vi "thscan_comparator_pix25.vi"() -> ()   [LabVIEW 2022 SP3]
panel:
  in  "Tab Control":enum32{"Single", "ROI"}(tab)
  out "Th Scan":u32[][](graph)=[[1, 1, 1, 1, 1, 1, 1, 1, 2, 71, 15005, 878042, 479272, 831838, 354879, 167379, 90908, 5540, 1668, 1480, 1359, 1170, 1144, 1050, 939, 886, 809, 720, 677, 630, 576, 523, 519, 483, 437, 402, 356, 337, 307, 320, 264, 275, 227, 222, 203, 176, 182, 179, 159, 135, 121, 110, 95, 105, 99, 71, 94, 91, 67, 61, 58, 55, 48, 31, 24, 26, 23, 15, 23, 17, 9, 11, 7, 5, 5, 4, 3, 3, 3, 1, 2, 2, 0, 1, 0, 0, 1, 0, 0, 1, 1, 0, 1, 1, 0, 0, 0, 0, 0, 0, 0], [1, 1, 1, 1, 1, 1, 1, 1, 2, 113, 14536, 860293, 575187, 892530, 326807, 156931, 85898, 3891, 481, 322, 328, 309, 273, 253, 234, 196, 206, 205, 157, 166, 143, 168, 135, 110, 116, 106, 90, 92, 74, 96, 70, 63, 73, 60, 55, 53, 50, 39, 38, 43, 33, 32, 28, 28, 21, 27, 19, 19, 15, 9, 10, 10, 10, 8, 8, 7, 5, 5, 10, 8, 6, 3, 2, 2, 0, 1, 1, 1, 0, 0, 0, 1, 1, 1, 0, 0, 0, 0, 0, 1, 0, 0, 0, 0, 0, 0, 0, 0, 0, 0, 0]]
  out "ThScans_Family":u32[][](graph)
  in  "Current File":u16(ring) items=["RED", "BLUE"]
  in  "file blue":path=path "C:/Users/User/OneDrive/measurements/pix25/PIX25/17_04_2023/M1/1_CountRate_gate_1s_iKRUM_14_setting_1/TS_step_10/itube_020_0417_101556"
  in  "file red":path=path "C:/Users/User/OneDrive/measurements/pix25/PIX25/17_04_2023/M1/1_CountRate_gate_1s_iKRUM_14_setting_1/TS_step_10/itube_080_0417_100615"
  out "MainImg":u32[][](graph)
  in  "ThScan_Load":bool
  in  "Exit":bool
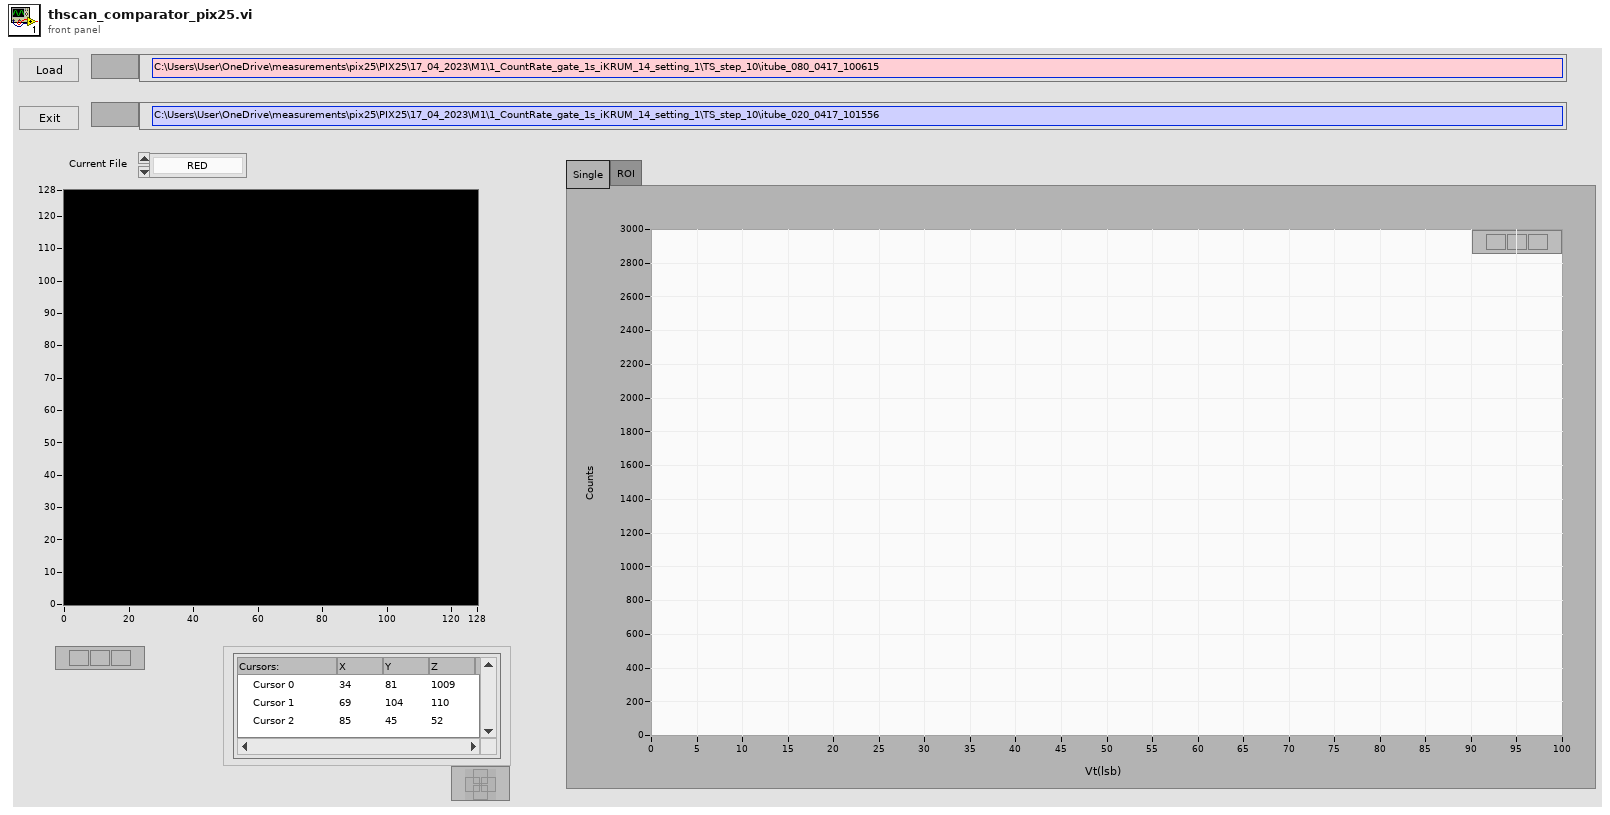
[diagram p1: front panel]
types:
  T1 = typedef "LVPointDoubleTypeDef.ctl" = cluster{"Cursor X":dbl, "Cursor Y":dbl}
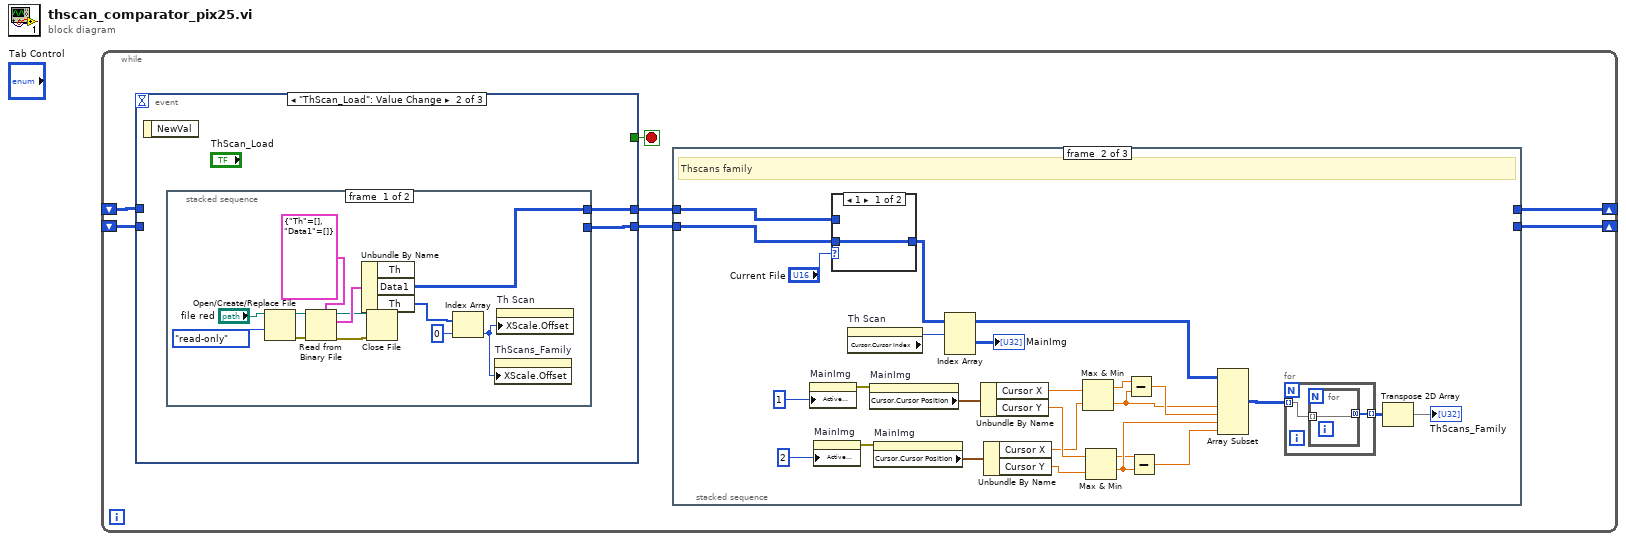
[diagram p0: block diagram]
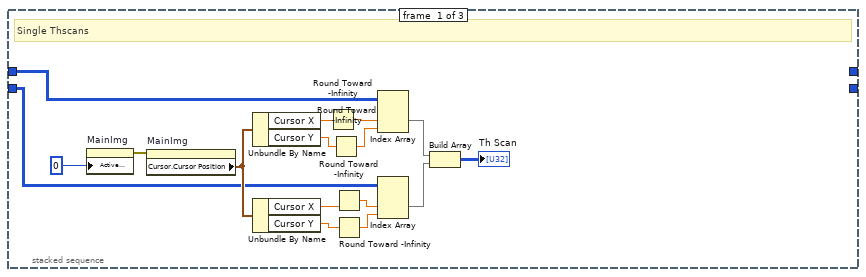
[diagram p2: hidden frame]
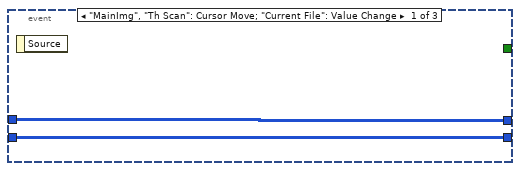
[diagram p5: hidden frame]
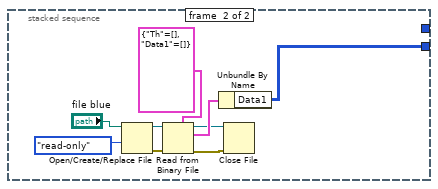
[diagram p6: hidden frame]
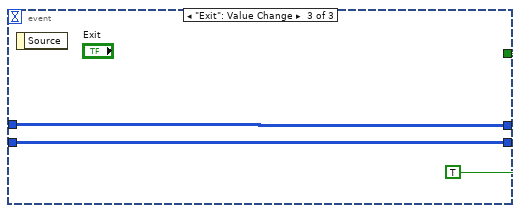
[diagram p7: hidden frame]
diagram:
  n1 = while {
    shift-right: [w1] -> _
    shift-left: _ -> [w6]
    shift-right: [w2] -> _
    shift-left: _ -> [w5]
    stop <- w7 stop-if-true
    n2 = event shown="[1] \"ThScan_Load\": Value Change" {
      selector: _ -> [_ _ _]
      dyn-events: _ -> [_ _ _]
      timeout: _ -> [_ _ _]
      tunnel: [_ _ TRUE] -> w7
      tunnel: w6 -> [w57 _ w82]
      tunnel: [w57 w59 w82] -> w4
      tunnel: [w56 w58 w81] -> w3
      tunnel: w5 -> [w56 _ w81]
      event "MainImg", "Th Scan": Cursor Move; "Current File": Value Change {
        n3 = event-data() -> ()  [unwired: 1 in, 1 out]
      }
      event "ThScan_Load": Value Change {
        n4 = event-data() -> ()  [unwired: 1 in, 1 out]
        n5 = stacked-sequence {
          tunnel: [_ w72] -> w59
          tunnel: [w60 _] -> w58
          frame #0 {
            n6 = Open/Create/Replace File(file path (use dialog)="file red", access (0:read/write)=enum16{"read/write", "read-only", "write-only"}."read-only") -> (refnum out=w68:refnum<file>, error out=w67:errorcluster)  [unwired: 4 in, 1 out]
            n7 = Read from Binary File(5:cluster{"Th":u16[], "Data1":u32[][][]} {"Th"=[], "Data1"=[]} ("TH Gate Scan"), 8:w67, 11:w68) -> (0:w70:errorcluster, 2:w71:cluster{"Th":u16[], "Data1":u32[][][]}, 3:w69:refnum<file>)  [unwired: 3 in, 1 out]
            n8 = Unbundle By Name(w71) -> ("Data1"=w60:u32[][][], "Th"=w61:u16[])  [unwired: 1 out]
            n9 = Close File(refnum=w69, error in=w70) -> ()  [unwired: 2 out]
            n10 = Index Array(array=w61, index=0) -> (element=w62:u16)
            n11 = property on="ThScans_Family" class="WFGraph (strict)"("XScale.Offset"=w62) -> ()  [unwired: 2 in, 2 out]
            n12 = property on="Th Scan" class="WFGraph (strict)"("XScale.Offset"=w62) -> ()  [unwired: 2 in, 2 out]
          }
          frame #1 {
            n13 = Open/Create/Replace File(file path (use dialog)="file blue", access (0:read/write)=enum16{"read/write", "read-only", "write-only"}."read-only") -> (refnum out=w77:refnum<file>, error out=w76:errorcluster)  [unwired: 4 in, 1 out]
            n14 = Read from Binary File(5:cluster{"Th":u16[], "Data1":u32[][][]} {"Th"=[], "Data1"=[]} ("TH Gate Scan"), 8:w76, 11:w77) -> (0:w79:errorcluster, 2:w80:cluster{"Th":u16[], "Data1":u32[][][]}, 3:w78:refnum<file>)  [unwired: 3 in, 1 out]
            n15 = Unbundle By Name(w80) -> ("Data1"=w72:u32[][][])
            n16 = Close File(refnum=w78, error in=w79) -> ()  [unwired: 2 out]
          }
        }
      }
      event "Exit": Value Change {
        n17 = event-data() -> ()  [unwired: 1 in, 1 out]
      }
    }
    n18 = stacked-sequence {
      tunnel: w4 -> [w8 w24 w54]
      tunnel: w3 -> [w9 w25 w55]
      tunnel: [_ _ w55] -> w2
      tunnel: [_ _ w54] -> w1
      frame #0 {
        # "Single Thscans"
        n19 = property on="MainImg" class="IntGraph (strict)"("Active Cursor"=u32 0) -> (error out=w11:errorcluster)  [unwired: 2 in, 1 out]
        n20 = property on="MainImg" class="IntGraph (strict)"(error in=w11) -> ("Cursor.Cursor Position"=w12:T1)  [unwired: 1 in, 2 out]
        n21 = Unbundle By Name(w12) -> ("Cursor X"=w21:dbl, "Cursor Y"=w22:dbl)
        n22 = Unbundle By Name(w12) -> ("Cursor X"=w17:dbl, "Cursor Y"=w18:dbl)
        n23 = Round Toward -Infinity(1:w21) -> (0:w20:dbl)
        n24 = Round Toward -Infinity(1:w22) -> (0:w23:dbl)
        n25 = Round Toward -Infinity(1:w17) -> (0:w16:dbl)
        n26 = Round Toward -Infinity(1:w18) -> (0:w19:dbl)
        n27 = Index Array(array=w9, index (dim 1)=w20, index (dim 2)=w23) -> (element=w15:u32[])  [unwired: 1 in]
        n28 = Index Array(array=w8, index (dim 1)=w16, index (dim 2)=w19) -> (element=w14:u32[])  [unwired: 1 in]
        n29 = Build Array(w15, w14) -> (→"Th Scan":u32[][])
      }
      frame #1 {
        # "Thscans family"
        n30 = property on="MainImg" class="IntGraph (strict)"("Active Cursor"=u32 1) -> (error out=w33:errorcluster)  [unwired: 2 in, 1 out]
        n31 = property on="MainImg" class="IntGraph (strict)"("Active Cursor"=u32 2) -> (error out=w34:errorcluster)  [unwired: 2 in, 1 out]
        n32 = case shown="1" "Current File" {
          tunnel: w25 -> [_ w53]
          tunnel: w24 -> [w52 _]
          tunnel: [w52 w53] -> w47
          frame 1 {
          }
          frame 0, Default {
          }
        }
        n33 = property on="Th Scan" class="WFGraph (strict)"() -> ("Cursor.Cursor Index"=w29:i32)  [unwired: 2 in, 2 out]
        n34 = property on="MainImg" class="IntGraph (strict)"(error in=w33) -> ("Cursor.Cursor Position"=w35:T1)  [unwired: 1 in, 2 out]
        n35 = property on="MainImg" class="IntGraph (strict)"(error in=w34) -> ("Cursor.Cursor Position"=w36:T1)  [unwired: 1 in, 2 out]
        n36 = Index Array(array=w47, index (dim 0)=w29) -> (element=→"MainImg":u32[][])  [unwired: 2 in]
        n37 = Unbundle By Name(w35) -> ("Cursor X"=w37:dbl, "Cursor Y"=w39:dbl)
        n38 = Unbundle By Name(w36) -> ("Cursor X"=w38:dbl, "Cursor Y"=w40:dbl)
        n39 = Max & Min(x=w37, y=w38) -> (max(x,y)=w41:dbl, min(x,y)=w42:dbl)
        n40 = Max & Min(x=w39, y=w40) -> (max(x,y)=w44:dbl, min(x,y)=w46:dbl)
        n41 = Subtract(x=w41, y=w42) -> (x-y=w43:dbl)
        n42 = Subtract(x=w44, y=w46) -> (x-y=w45:dbl)
        n43 = Array Subset(array=w47, index (dim 1)=w42, length (dim 1)=w43, index (dim 2)=w46, length (dim 2)=w45) -> (w31:u32[][][])  [unwired: 2 in]
        n44 = for {
          tunnel: [w50] -> w30 mode=indexing
          tunnel: w31 -> [w49] mode=indexing
          n45 = for {
            tunnel: w49 -> [w51] mode=indexing
            tunnel: [w51] -> w50 mode=concatenating
          }
        }
        n46 = Transpose 2D Array(2D array=w30) -> (transposed array=→"ThScans_Family":u32[][])
      }
      frame #2 {
      }
    }
  }
